vi "UI SaveAs Config.vi"(8 "error in (no error)":errorcluster, 11 "UI_Left_Right in":refnum<class "UI_Left_Right.lvclass">) -> (0 "error out":errorcluster, 3 "UI_Left_Right out":refnum<class "UI_Left_Right.lvclass">)   [LabVIEW 2021, in "UI_Left_Right.lvclass"]
uses:
  UI_Left_Right.lvclass
  <userlib>/John_Lib/AbstractActorTemplate/AbstractActorTemplate/UIActorTop.lvclass
  UI_Left_Right.lvclass/UI_Left_Right.ctl
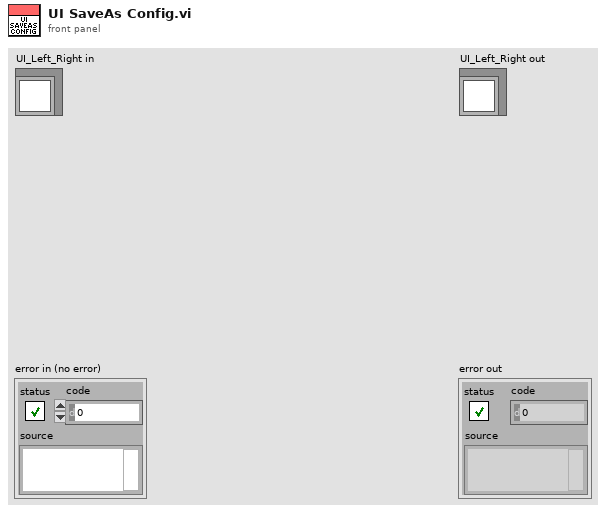
[diagram p1: front panel]
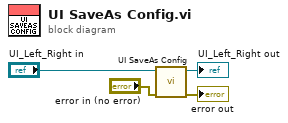
[diagram p0: block diagram]
diagram:
  n1 = call-parent "UI SaveAs Config.vi"("error in (no error)"="error in (no error)", "UIActorTop in"="UI_Left_Right in") -> ("error out"=→"error out":errorcluster, "UIActorTop out"=→"UI_Left_Right out":refnum<class "UI_Left_Right.lvclass">)  [unwired: 8 in]
